vi "Draw Layers.vi"(11 "Display State In in":T1 caption="State") -> (3 "Display State In out":T1 caption="State")   [LabVIEW 2016, in "Horizontal MenuList.xctl"]
uses:
  Horizontal MenuList.xctl
  Horizontal MenuList_State.ctl
  Highlight Colors.ctl
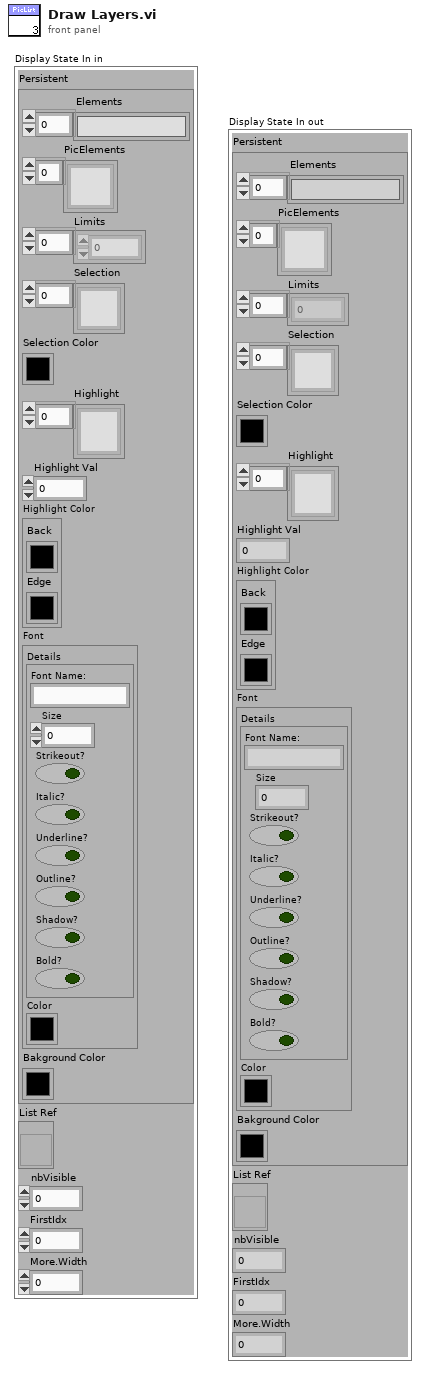
[diagram p1: front panel]
types:
  T1 = typedef "Horizontal MenuList.xctl/Horizontal MenuList_State.ctl" = cluster{"Persistent":cluster{"Elements":string[], "PicElements":picture[], "Limits":i32[], "Selection":picture[], "Selection Color":u32, "Highlight":picture[], "Highlight Val":i32, "Highlight Color":T2, "Font":cluster{"Details":cluster{"Font Name:":string, "Size":i16, "Strikeout?":bool, "Italic?":bool, "Underline?":bool, "Outline?":bool, "Shadow?":bool, "Bold?":bool}, "Color":u32}, "Bakground Color":u32}, "List Ref":refnum<vi>, "nbVisible":u8, "FirstIdx":u8, "More.Width":u8}
  T2 = typedef "Horizontal MenuList.xctl/Highlight Colors.ctl" = cluster{"Back":u32, "Edge":u32}
  T3 = enum16{"User-specified Font", "Application Font", "System Font", "Dialog Font"}
  T4 = cluster{"horizontal":enum16{"left", "center", "right"}, "vertical":enum16{"top", "center", "bottom"}}
  T5 = cluster{"Details":cluster{"Font Name:":string, "Size":i16, "Strikeout?":bool, "Italic?":bool, "Underline?":bool, "Outline?":bool, "Shadow?":bool, "Bold?":bool}, "Color":u32}
  T6 = typedef "LVBoundsTypeDef.ctl" = cluster{"Width":u32, "Height":u32}
  T7 = cluster{"Font Name:":string, "Size":i16, "Strikeout?":bool, "Italic?":bool, "Underline?":bool, "Outline?":bool, "Shadow?":bool, "Bold?":bool}
  T8 = cluster{"left":i16, "top":i16, "right":i16, "bottom":i16}
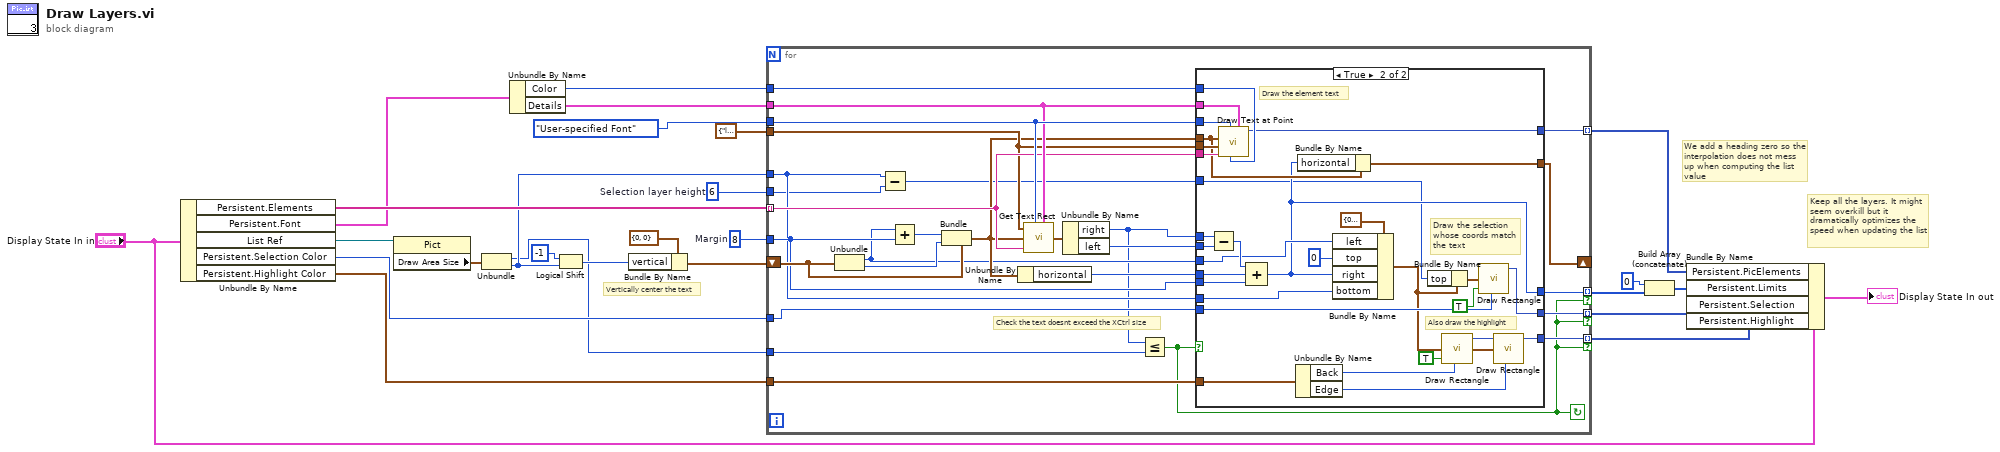
[diagram p0: block diagram]
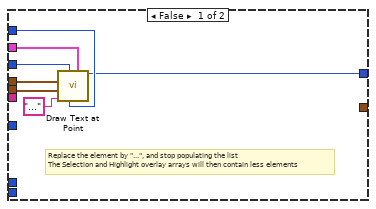
[diagram p2: hidden frame]
diagram:
  w1 = u32 6  # Selection layer height
  w11 = 8  # Margin
  # "We add a heading zero so the interpolation does not mess up when computing the list value"
  # "Keep all the layers. It might seem overkill but it dramatically optimizes the speed when updating the list"
  # "Vertically center the text"
  n1 = Unbundle By Name("Display State In in") -> ("Persistent.Elements"=w26:string[], "Persistent.Font"=w23:T5, "List Ref"=w13:refnum<vi>, "Persistent.Selection Color"=w16:u32, "Persistent.Highlight Color"=w15:T2)
  n2 = property class="Pict"(reference=w13) -> ("Draw Area Size"=w6:T6)  [unwired: 1 in, 2 out]
  n3 = Unbundle(w6) -> ("Width"=w3:u32, "Height"=w12:u32)
  n4 = Unbundle By Name(w23) -> ("Color"=w24:u32, "Details"=w2:T7)
  n5 = Logical Shift(y=i16 -1, x=w12) -> (x << y=w10:u32)
  n6 = Bundle By Name(cluster=cluster{"horizontal":i16, "vertical":i16} {"horizontal"=0, "vertical"=0} ("origin(0,0)"), "vertical"=w10) -> (w14:cluster{"horizontal":i16, "vertical":i16})
  n7 = for {
    tunnel: T3."User-specified Font" ("Mode") -> [w53]
    tunnel: w2 -> [w52]
    tunnel: w24 -> [w51]
    tunnel: w26 -> [w50] mode=indexing
    tunnel: [w49] -> w17 mode=indexing
    tunnel: T4 {"horizontal"=enum."left", "vertical"=enum."center"} ("alignment(left, top)") -> [w48]
    shift-right: [w42] -> _
    shift-left: w14 -> [w44]
    tunnel: w11 -> [w41]
    tunnel: [w47] -> w22 mode=indexing if=w28
    tunnel: w12 -> [w31]
    tunnel: [w35] -> w18 mode=indexing if=w28
    tunnel: [w37] -> w21 mode=indexing if=w28
    tunnel: w15 -> [w32]
    tunnel: w16 -> [w33]
    tunnel: w3 -> [w29]
    tunnel: w1 -> [w27]
    stop <- w28 continue-if-true
    # "Check the text doesnt exceed the XCtrl size"
    n8 = Unbundle(w44) -> ("horizontal"=w36:i16, "vertical"=w39:i16)
    n9 = Subtract(x=w31, y=w27) -> (x-y=w34:u32)
    n10 = Add(x=w36, y=w41) -> (x+y=w43:i32)
    n11 = Bundle(cluster=w44, "horizontal"=w43, "vertical"=w39) -> (w38:cluster{"horizontal":i16, "vertical":i16})
    n12 = Unbundle By Name(w38) -> ("horizontal"=w40:i16)
    n13 = call <vilib>:"Get Text Rect.vi"("alignment(left, top)"=w48, "desired font(Application)"=w53, "origin(0,0)"=w38, "text"=w50, "[user-specified font]"=w52) -> ("rect"=w45:T8)  [unwired: 4 in]
    n14 = Unbundle By Name(w45) -> ("right"=w30:i16, "left"=w46:i16)
    n15 = Less Or Equal?(x=w30, y=w29) -> (x <= y?=w28:bool)
    n16 = case shown="True" w28 {
      tunnel: w53 -> [w59 w90]
      tunnel: w52 -> [w60 w89]
      tunnel: w51 -> [w58 w88]
      tunnel: w50 -> [_ w87]
      tunnel: [w54 w86] -> w49
      tunnel: w48 -> [w56 w84]
      tunnel: [_ w83] -> w47
      tunnel: w46 -> [_ w81]
      tunnel: [_ w80] -> w42
      tunnel: w41 -> [_ w79]
      tunnel: w40 -> [_ w78]
      tunnel: w38 -> [w55 w77]
      tunnel: [_ w76] -> w37
      tunnel: w36 -> [_ w74]
      tunnel: [_ w73] -> w35
      tunnel: w34 -> [_ w72]
      tunnel: w33 -> [_ w70]
      tunnel: w32 -> [_ w69]
      tunnel: w31 -> [_ w63]
      tunnel: w30 -> [_ w61]
      frame False {
        # "Replace the element by \"...\", and stop populating the list\nThe Selection and Highlight overlay arrays will then contain less elements"
        n17 = call <vilib>:"Draw Text at Point.vi"("[user-specified font]"=w60, "text color(black)"=w58, "desired font(Application)"=w59, "text"="...", "alignment(left, top)"=w56, "origin"=w55) -> ("new picture"=w54:picture)  [unwired: 4 in, 1 out]
      }
      frame True {
        # "Also draw the highlight"
        # "Draw the selection whose coords match the text"
        # "Draw the element text"
        n18 = Subtract(x=w61, y=w81) -> (x-y=w85:i16)
        n19 = call <vilib>:"Draw Text at Point.vi"("[user-specified font]"=w89, "text color(black)"=w88, "desired font(Application)"=w90, "text"=w87, "alignment(left, top)"=w84, "origin"=w77) -> ("new picture"=w86:picture)  [unwired: 4 in, 1 out]
        n20 = Compound Arithmetic op=unknown(w85, w78, w79) -> (w73:i32)
        n21 = Unbundle By Name(w69) -> ("Back"=w65:u32, "Edge"=w64:u32)
        n22 = Bundle By Name(cluster=w77, "horizontal"=w73) -> (w80:cluster{"horizontal":i16, "vertical":i16})
        n23 = Bundle By Name(cluster=T8 {"left"=0, "top"=0, "right"=0, "bottom"=0} ("rect"), "left"=w74, "top"=i16 0, "right"=w73, "bottom"=w63) -> (w66:T8)
        n24 = Bundle By Name(cluster=w66, "top"=w72) -> (w71:T8)
        n25 = call <vilib>:"Draw Rectangle.vi"("rect"=w66, "fill?(F)"=TRUE, "color(black)"=w65) -> ("new picture"=w67:picture)  [unwired: 6 in]
        n26 = call <vilib>:"Draw Rectangle.vi"("rect"=w71, "fill?(F)"=TRUE, "color(black)"=w70) -> ("new picture"=w76:picture)  [unwired: 6 in]
        n27 = call <vilib>:"Draw Rectangle.vi"("picture"=w67, "rect"=w66, "color(black)"=w64) -> ("new picture"=w83:picture)  [unwired: 6 in]
      }
    }
  }
  n28 = Build Array (concatenate)(0 ("y"), w18) -> (w20:i32[])
  n29 = Bundle By Name(cluster="Display State In in", "Persistent.PicElements"=w17, "Persistent.Limits"=w20, "Persistent.Selection"=w21, "Persistent.Highlight"=w22) -> (→"Display State In out":T1)
